vi "LineFollower.vi"() -> ()   [LabVIEW 2016]
uses:
  <vilib>/NXT/Block Support/NXT_InputPort.ctl
  <vilib>/NXT/Subs/MotorOutput.ctl
  <vilib>/NXT/Dual Mode Library/Sensors/Light_On.vi
  <vilib>/NXT/Dual Mode Library/Motors/MotorOn.vi
panel:
  in  "Base Speed":i16
  in  "Gain":i16
  in  "Centered Value":i16
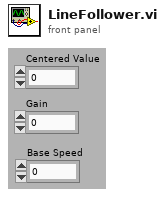
[diagram p1: front panel]
types:
  T1 = typedef "MotorOutput.ctl" = u8
  T2 = typedef "NXT_InputPort.ctl" = u32
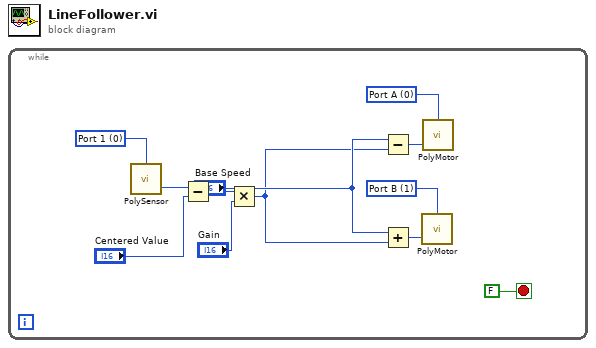
[diagram p0: block diagram]
diagram:
  n1 = while {
    stop <- FALSE stop-if-true
    w3 = T1 1 items=["Port A"=0, "Port B"=1, "Port C"=2, "Ports A & B"=4, "Ports A & C"=5, "Ports B & C"=6, "All Ports"=3] ("Output Port (All Ports)")
    w4 = T1 0 items=["Port A"=0, "Port B"=1, "Port C"=2, "Ports A & B"=4, "Ports A & C"=5, "Ports B & C"=6, "All Ports"=3] ("Output Port (All Ports)")
    w5 = T2 0 items=["Port 1", "Port 2", "Port 3", "Port 4"] ("Port (Port 3)")
    n2 = call-poly <vilib>:"PolySensor.vi"("Port (Port 3)"=w5) -> ("Scaled Value"=w11:i16)  [unwired: 2 in, 1 out]
    n3 = Subtract(x=w11, y="Centered Value") -> (x-y=w9:i16)
    n4 = Multiply(x=w9, y="Gain") -> (x*y=w1:i16)
    n5 = Subtract(x="Base Speed", y=w1) -> (x-y=w7:i16)
    n6 = Add(x="Base Speed", y=w1) -> (x+y=w6:i16)
    n7 = call-poly <vilib>:"PolyMotor.vi"("Power (75)"=w6, "Output Port (All Ports)"=w3) -> ()  [unwired: 2 in, 1 out]
    n8 = call-poly <vilib>:"PolyMotor.vi"("Power (75)"=w7, "Output Port (All Ports)"=w4) -> ()  [unwired: 2 in, 1 out]
  }
